vi "labviewtcrt5000IR.vi"() -> ()   [LabVIEW 2018]
uses:
  <vilib>/MakerHub/LINX/Public/Peripherals/Analog/Analog Read 1 Chan.vi
  <vilib>/MakerHub/LINX/Public/Peripherals/Digital/Digital Read 1 Chan.vi
  <vilib>/MakerHub/LINX/Public/Peripherals/Analog/Analog Read N Chans.vi
  <vilib>/MakerHub/LINX/Public/Peripherals/Digital/Digital Read N Chans.vi
  <vilib>/MakerHub/LINX/Private/Local IO/LinxAnalogRead.vi
  <vilib>/MakerHub/LINX/Public/Utilities/Check Channel.vi
  <vilib>/MakerHub/LINX/Private/Local IO/LinxDigitalRead.vi
  <vilib>/MakerHub/LINX/Public/Utilities/Open Serial.vi
  <vilib>/MakerHub/LINX/Private/Utilties/Generate Error.vi
  <vilib>/smtpClient/Set Message Text.vi
  <vilib>/MakerHub/LINX/LMH-LINX.lvlib
  <vilib>/smtpClient/LabVIEWSMTPClient.lvlib
panel:
  out "MAİL GÖNDERİLDİ":bool
  out "TESPİT ADET":dbl(knob) scale=0.0..500.0
  out "Voltage Waveform Chart":dbl(graph)
  out "Analog Ref Override (V)":dbl
  out "Voltage":dbl
  in  "TCRT5000 SENSÖR PİN":u8
  in  "Error In":errorcluster
  in  "Baud Rate Override":u32
  in  "Serial Port":refnum<visa-resource-name>="N/A"
  out "TESPİT ADET":dbl
  in  "STOP":bool
  out "TESPİT":bool
  # "EMRE BURAK EL"
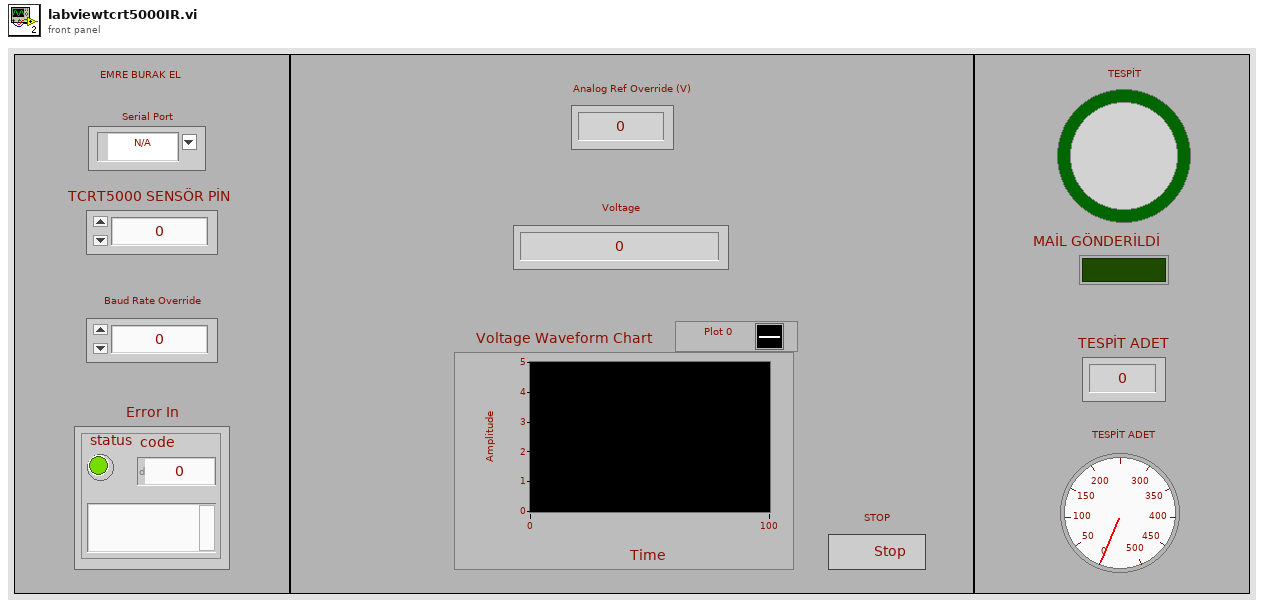
[diagram p1: front panel]
types:
  T1 = typedef "LMH-LINX.lvlib/LINX Ref.ctl" = cluster{"IO":T2, "Interface":T3, "LINX Device Config":T4}
  T2 = typedef "LMH-LINX.lvlib/Platform.ctl" = enum16{"Remote", "Local"}
  T3 = typedef "LMH-LINX.lvlib/Interface.ctl" = enum16{"Serial", "TCP"}
  T4 = typedef "LMH-LINX.lvlib/Device.lvlib/LINX Device Config.ctl" = cluster{"Interface":T3, "COM Port":refnum<visa-resource-name>, "TCP Configuration":T5, "Device Family":u8, "Device ID":u8, "Device Name":string, "TCP Ref":refnum<k5>, "Channels":T6}
  T5 = typedef "LMH-LINX.lvlib/Device.lvlib/TCP Config.ctl" = cluster{"IP Address":string, "Port":u16}
  T6 = typedef "LMH-LINX.lvlib/Channels.ctl" = cluster{"DI":u8[], "DO":u8[], "AI":u8[], "AO":u8[], "PWM":u8[], "QE":u8[], "UART":u8[], "I2C 2":u8[], "SPI":u8[], "CAN":u8[], "Servo":u8[], "AI Ref (V)":dbl, "AI Resolution (Bits)":u8, "AO Ref (V)":dbl, "AO Resolution (Bits)":u8}
  T7 = typedef "LabVIEWSMTPClient.lvlib/SmtpClientHandle.ctl" = refnum<k1>
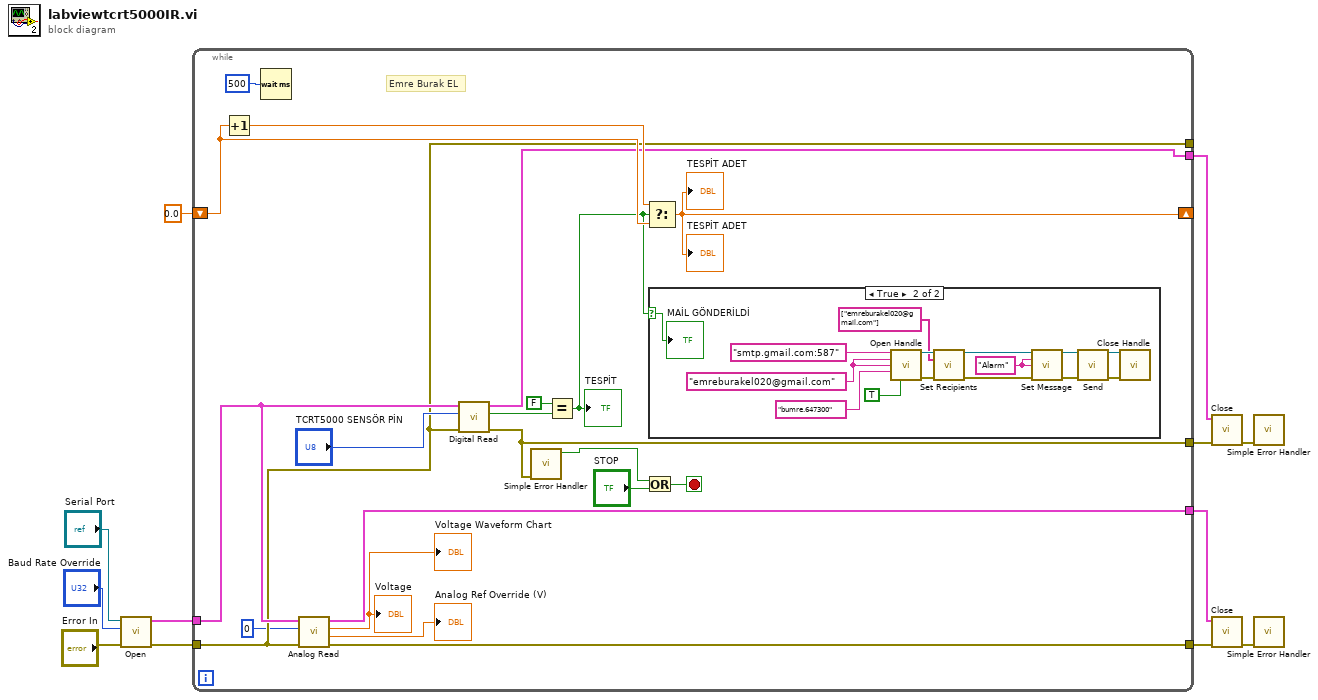
[diagram p0: block diagram]
diagram:
  n1 = call-poly <vilib>:"Open.vi"("Error In"="Error In", "Baud Rate Override"="Baud Rate Override", "Serial Port"="Serial Port") -> ("Error Out"=w11:errorcluster, "LINX Resource"=w12:T1)  [unwired: 6 in, 1 out]
  n2 = while {
    tunnel: w12 -> [w21]
    tunnel: [w20] -> _
    tunnel: w11 -> [w20]
    tunnel: [w27] -> w10
    tunnel: [w29] -> w2
    shift-right: [w14] -> _
    shift-left: 0.0 -> [w31]
    tunnel: [w19] -> w4
    tunnel: [w18] -> w3
    stop <- w24 stop-if-true
    # "Emre Burak EL"
    n3 = Increment(x=w31) -> (x+1=w32:dbl)
    n4 = Wait (ms)(milliseconds to wait=u32 500) -> ()  [unwired: 1 out]
    n5 = call-poly <vilib>:"Analog Read.vi"("Error In"=w20, "Analog Channel"=u8 0, "LINX Resource"=w21) -> ("Error Out"=w18:errorcluster, "AI Ref"=→"Analog Ref Override (V)":dbl, "Voltage"=→"Voltage" →"Voltage Waveform Chart":dbl, "LINX Resource"=w19:T1)  [unwired: 5 in]
    n6 = call-poly <vilib>:"Digital Read.vi"("Error In"=w20, "DI Channel"="TCRT5000 SENSÖR PİN", "LINX Resource"=w21) -> ("Error Out"=w27:errorcluster, "DI Value"=w28:bool, "LINX Resource"=w29:T1)  [unwired: 6 in]
    n7 = call <vilib>:"Simple Error Handler.vi"("error in (no error)"=w27) -> ("error?"=w25:bool)  [unwired: 4 in, 4 out]
    n8 = Equal?(x=FALSE, y=w28) -> (x = y?=w13:bool)
    "TESPİT" <- w13
    n9 = Or(x=w25, y="STOP") -> (x .or. y?=w24:bool)
    n10 = Select(t=w32, s=w13, f=w31) -> (s? t:f=w14:dbl)
    "TESPİT ADET" <- w14
    "TESPİT ADET" <- w14
    n11 = case shown="True" w13 {
      selector: w13 -> [_ w33]
      frame False {
      }
      frame True {
        w39 = "Alarm" ("subject")
        w36 = "emreburakel020@gmail.com" ("from")
        n12 = call <vilib>:"Open Handle.vi"("server address"="smtp.gmail.com:587", "from"=w36, "username"=w36, "password"="bumre.647300", "use TLS (false)"=TRUE) -> ("handle out"=w45:T7, "error out"=w44:errorcluster)  [unwired: 9 in]
        n13 = call <vilib>:"Set Recipients.vi"("handle in"=w45, "to"=string[] ["emreburakel020@gmail.com"], "error in (no error)"=w44) -> ("handle out"=w43:T7, "error out"=w42:errorcluster)  [unwired: 11 in]
        n14 = call-poly <vilib>:"Set Message.vi"("handle in"=w43, "subject"=w39, "plain text message"=w39, "error in (no error)"=w42) -> ("handle out"=w41:T7, "error out"=w40:errorcluster)  [unwired: 10 in]
        n15 = call <vilib>:"Send.vi"("handle in"=w41, "error in (no error)"=w40) -> ("handle out"=w46:T7, "error out"=w47:errorcluster)  [unwired: 11 in, 1 out]
        n16 = call <vilib>:"Close Handle.vi"("handle in"=w46, "error in (no error)"=w47) -> ()  [unwired: 12 in, 2 out]
        "MAİL GÖNDERİLDİ" <- w33
      }
    }
  }
  n17 = call <vilib>:"Close.vi"("Error In"=w10, "LINX Resource"=w2) -> ("Error Out"=w8:errorcluster)  [unwired: 9 in]
  n18 = call <vilib>:"Close.vi"("Error In"=w3, "LINX Resource"=w4) -> ("Error Out"=w1:errorcluster)  [unwired: 9 in]
  n19 = call <vilib>:"Simple Error Handler.vi"("error in (no error)"=w8) -> ()  [unwired: 4 in, 5 out]
  n20 = call <vilib>:"Simple Error Handler.vi"("error in (no error)"=w1) -> ()  [unwired: 4 in, 5 out]
